vi "倒计时.vi"() -> ()   [LabVIEW 2017]
panel:
  in  "开始倒计时":bool
  in  "定时时间选择":enum16{"6", "10", "20"}(ring)
  out "倒计时":string
  out "?":bool
  in  "停止":bool
  # "倒计时"
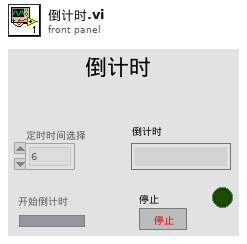
[diagram p1: front panel]
types:
  T1 = enum8{"Enabled", "Disabled", "Disabled and Grayed Out"}
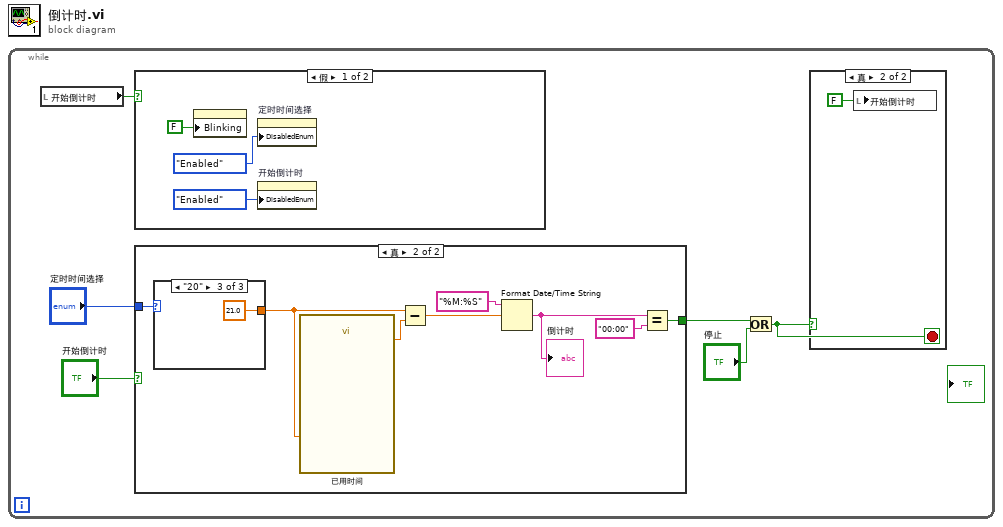
[diagram p0: block diagram]
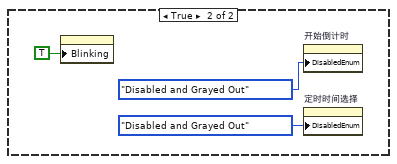
[diagram p3: hidden frame]
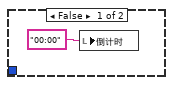
[diagram p4: hidden frame]
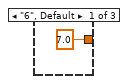
[diagram p5: hidden frame]
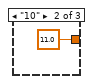
[diagram p6: hidden frame]
diagram:
  n1 = while {
    stop <- w1 stop-if-true
    n2 = local read "开始倒计时"() -> (w3:bool)
    n3 = case shown="假" w3 {
      frame False {
        n4 = property class="Bool (严格)"("Blinking"=FALSE ("闪烁")) -> ()  [unwired: 2 in, 2 out]
        n5 = property on="定时时间选择" class="Enum (严格)"("DisabledEnum"=T1."Enabled" ("禁用")) -> ()  [unwired: 2 in, 2 out]
        n6 = property on="开始倒计时" class="Bool (严格)"("DisabledEnum"=T1."Enabled" ("禁用")) -> ()  [unwired: 2 in, 2 out]
      }
      frame True {
        n7 = property class="Bool (严格)"("Blinking"=TRUE ("闪烁")) -> ()  [unwired: 2 in, 2 out]
        n8 = property on="开始倒计时" class="Bool (严格)"("DisabledEnum"=T1."Disabled and Grayed Out" ("禁用")) -> ()  [unwired: 2 in, 2 out]
        n9 = property on="定时时间选择" class="Enum (严格)"("DisabledEnum"=T1."Disabled and Grayed Out" ("禁用")) -> ()  [unwired: 2 in, 2 out]
      }
    }
    n10 = case shown="真" "开始倒计时" {
      tunnel: [_ w15] -> w2
      tunnel: "定时时间选择" -> [_ w16]
      frame False {
        n11 = local write "倒计时"("00:00" ("倒计时")) -> ()
      }
      frame True {
        n12 = case shown="\"20\"" w16 {
          tunnel: [7.0 ("Time Target (s)") 11.0 ("Time Target (s)") 21.0 ("Time Target (s)")] -> w21
          frame "6", Default {
          }
          frame "10" {
          }
          frame "20" {
          }
        }
        n13 = call "已用时间"("Time Target (s)"=w21) -> ("Elapsed Time (s)"=w20:dbl)  [unwired: 11 in, 7 out]
        n14 = Subtract(x=w21, y=w20) -> (x-y=w19:dbl)
        n15 = Format Date/Time String ("格式化日期/时间字符串")(time format string (%c)="%M:%S" ("时间格式字符串(%c)"), seconds (now)=w19) -> (date/time string=w18:string)  [unwired: 1 in]
        "倒计时" <- w18
        n16 = Equal?(x=w18, y="00:00" ("倒计时")) -> (x = y?=w15:bool)
      }
    }
    n17 = Or(x=w2, y="停止") -> (x .or. y?=w1:bool)
    n18 = case shown="真" w1 {
      frame False {
      }
      frame True {
        n19 = local write "开始倒计时"(FALSE ("开始倒计时")) -> ()
      }
    }
  }
